vi "05 - Optimised Image Loading.vi"() -> ()   [LabVIEW 2015]
uses:
  Libraries/LibSDL2 Wrapper/Controls/Rectangle.ctl
  Libraries/LibSDL2 Wrapper/Controls/Init Flags.ctl
  Libraries/LibSDL2 Wrapper/Controls/Surface.ctl
  <vilib>/Utility/importsl/GetValueByPointer/datatype.ctl
  Libraries/LibSDL2 Wrapper/Controls/NULL.ctl
  <vilib>/Utility/importsl/GetValueByPointer/GetValueByPointer.xnode
  Libraries/LibSDL2 Wrapper/LibSDL2.lvlib
  Libraries/SDL2 Utility/SDL2 Utility.lvlib
  Libraries/Win32 Util/Win32 Util.lvlib
panel:
  in  "Scale":bool
  in  "Destination Rectangle":T1={"x"=-123, "y"=-114, "Width"=553, "Height"=415}
  in  "Source Rectangle":T1={"x"=0, "y"=0, "Width"=622, "Height"=495}
  in  "stop":bool
  out "Error":string
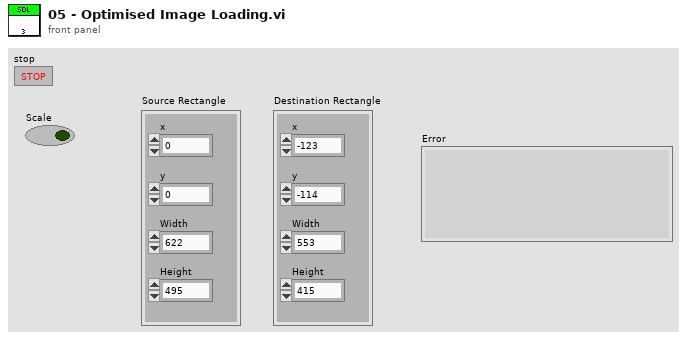
[diagram p1: front panel]
types:
  T1 = typedef "LibSDL2.lvlib/Rectangle.ctl" = cluster{"x":i32, "y":i32, "Width":i32, "Height":i32}
  T2 = enum32{"pack1", "pack2", "pack4", "pack8", "pack16"}
  T3 = typedef "LibSDL2.lvlib/Surface.ctl" = cluster{"Flags":u32, "Pixel Format Pointer":u32, "Width":i32, "Height":i32, "Pitch":i32, "Pixels Pointer":u32, "User Data Pointer":u32, "Locked":i32, "Lock Data Pointer":u32, "Clip Rectangle":T1, "Blitmap Pointer":u32, "Ref Count":i32}
  T4 = typedef "LibSDL2.lvlib/Init Flags.ctl" = u32
  T5 = typedef "LibSDL2.lvlib/NULL.ctl" = enum32{"NULL"}
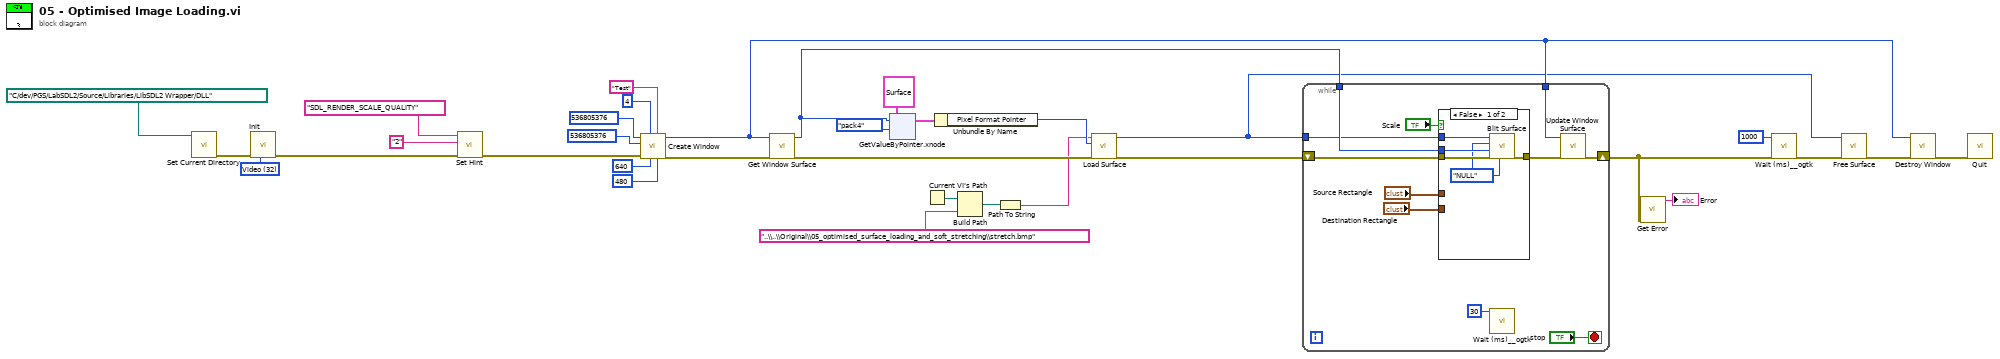
[diagram p0: block diagram]
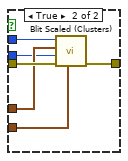
[diagram p2: hidden frame]
diagram:
  w33 = T4 32 items=["Timer"=1, "Audio"=16, "Video"=32, "Joystick"=512, "Haptic"=4096, "Game Controller"=8192, "Events"=16384, "No Parachute"=1048576, "Everything"=17244689] ("Init Flags")
  n1 = call "Set Current Directory.vi"("Path"=path "C:/dev/PGS/LabSDL2/Source/Libraries/LibSDL2 Wrapper/DLL" ("DLL Directory")) -> ("error out"=w6:errorcluster)  [unwired: 10 in]
  n2 = call "Init.vi"("Flags"=w33, "error in"=w6) -> ("error out"=w10:errorcluster)  [unwired: 8 in, 1 out]
  n3 = call "Set Hint.vi"("error in"=w10, "Value"="2", "Name"="SDL_RENDER_SCALE_QUALITY") -> ("error out"=w9:errorcluster)  [unwired: 7 in, 1 out]
  n4 = call "Create Window.vi"("Height"=480, "Title"="Test", "Width"=640, "Flags"=u32 4, "error in"=w9, "Position y"=u32 536805376 ("Flags"), "Position x"=u32 536805376 ("Flags")) -> ("error out"=w23:errorcluster, "Window Pointer"=w17:u32)  [unwired: 3 in]
  n5 = call "Get Window Surface.vi"("error in"=w23, "Window Pointer"=w17) -> ("error out"=w14:errorcluster, "Surface Pointer"=w16:u32)  [unwired: 8 in]
  n6 = xnode "GetValueByPointer.xnode"("Pointer"=w16, "InputType"=T3 {"Flags"=0, "Pixel Format Pointer"=0, "Width"=0, "Height"=0, "Pitch"=0, "Pixels Pointer"=0, "User Data Pointer"=0, "Locked"=0, "Lock Data Pointer"=0, "Clip Rectangle"={"x"=0, "y"=0, "Width"=0, "Height"=0}, "Blitmap Pointer"=0, "Ref Count"=0} ("Surface"), "PackType"=T2."pack4") -> ("Output"=w18:T3)  [unwired: 1 in, 1 out]
  n7 = Current VI's Path() -> (path=w2:path)
  n8 = Unbundle By Name(w18) -> ("Pixel Format Pointer"=w12:u32)
  n9 = Build Path(base path=w2, name or relative path="..\\..\\Original\\05_optimised_surface_loading_and_soft_stretching\\stretch.bmp" ("File")) -> (appended path=w3:path)
  n10 = Path To String(path=w3) -> (string=w1:string)
  n11 = call "Load Surface.vi"("error in"=w14, "Pixel Format Pointer"=w12, "File"=w1) -> ("error out"=w13:errorcluster, "Optimised Surface Pointer"=w11:u32)  [unwired: 7 in]
  n12 = while {
    tunnel: w17 -> [w44]
    tunnel: w16 -> [w43]
    tunnel: w11 -> [w42]
    shift-right: [w39] -> w15
    shift-left: w13 -> [w41]
    stop <- "stop" stop-if-true
    n13 = case shown="False" "Scale" {
      tunnel: w43 -> [w49 w51]
      tunnel: w42 -> [w48 w53]
      tunnel: w41 -> [w47 w55]
      tunnel: [w46 w54] -> w40
      tunnel: "Source Rectangle" -> [_ w52]
      tunnel: "Destination Rectangle" -> [_ w50]
      frame False {
        w45 = NULL."NULL" ("Null")
        n14 = call "Blit Surface.vi"("Destination Rectangle Pointer"=w45, "error in"=w47, "Destination Surface Pointer"=w49, "Source Rectangle Pointer"=w45, "Source Surface Pointer"=w48) -> ("error out"=w46:errorcluster)  [unwired: 5 in, 1 out]
      }
      frame True {
        n15 = call "Blit Scaled (Clusters).vi"("Destination Rectangle"=w50, "error in"=w55, "Destination Surface Pointer"=w51, "Source Rectangle"=w52, "Source Surface Pointer"=w53) -> ("error out"=w54:errorcluster)  [unwired: 5 in, 1 out]
      }
    }
    n16 = call <userlib>:"Wait (ms)__ogtk.vi"("milliseconds to wait"=u32 30) -> ()  [unwired: 9 in, 2 out]
    n17 = call "Update Window Surface.vi"("error in"=w40, "Window Pointer"=w44) -> ("error out"=w39:errorcluster)  [unwired: 9 in]
  }
  n18 = call "Get Error.vi"("error in"=w15) -> ("Error"=→"Error":string)  [unwired: 9 in, 1 out]
  n19 = call <userlib>:"Wait (ms)__ogtk.vi"("error in (no error)"=w15, "milliseconds to wait"=u32 1000) -> ("error out"=w22:errorcluster)  [unwired: 8 in, 1 out]
  n20 = call "Free Surface.vi"("error in"=w22, "Surface Pointer"=w11) -> ("error out"=w21:errorcluster)  [unwired: 9 in]
  n21 = call "Destroy Window.vi"("error in"=w21, "Window Pointer"=w17) -> ("error out"=w25:errorcluster)  [unwired: 9 in]
  n22 = call "Quit.vi"("error in"=w25) -> ()  [unwired: 10 in, 1 out]
